vi "Delete Int16 DVR.vi"(8 "error in (no error)":errorcluster, 11 "Int16 DVR in":refnum<data-value>) -> (0 "error out":errorcluster, 3 "Int16 out":refnum<class "Int16.lvclass">)   [LabVIEW 2012, in "MDSplus.lvlib" / "Int16.lvclass"]
uses:
  <vilib>/MDSplus/Classes/Data_Class/Scalar_Class/Int16_Class/Int16.lvclass
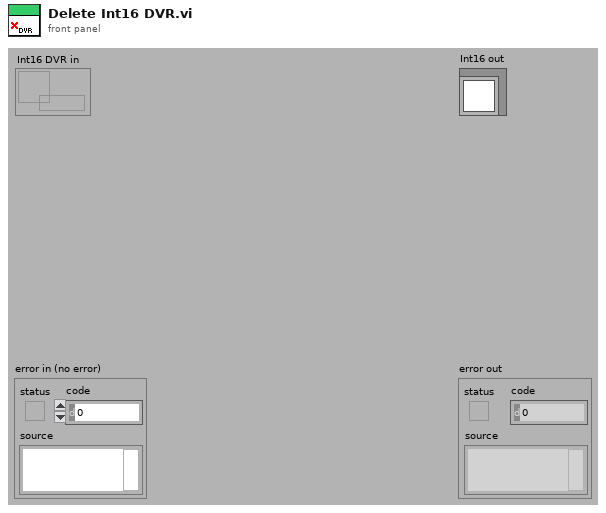
[diagram p1: front panel]
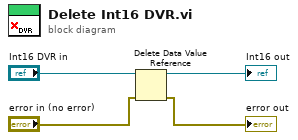
[diagram p0: block diagram]
diagram:
  n1 = Delete Data Value Reference(data value reference="Int16 DVR in", error in="error in (no error)") -> (data value=→"Int16 out":refnum<class "Int16.lvclass">, error out=→"error out":errorcluster)
